vi "CMD_AEROSCRIPTRUN.vi"(6 "Gantry in":refnum<class "Gantry.lvclass">, 8 "error in (no error)":errorcluster, 10 "Arguments":string[](array[string]), 11 "gScript Interpreter in":refnum<class "gScript Interpreter.lvclass">) -> (0 "error out":errorcluster, 3 "gScript Interpreter out":refnum<class "gScript Interpreter.lvclass">, 4 "Gantry out":refnum<class "Gantry.lvclass">)   [LabVIEW 2026, in "gScript Interpreter.lvclass"]
uses:
  gScript Interpreter.lvclass
  Shared Components/Gantry Class/Gantry.lvclass
  Shared Components/FlexWorktable/FlexWorktable.lvclass
  <instrlib>/Aerotech Automation1/Aerotech Automation1.lvlib
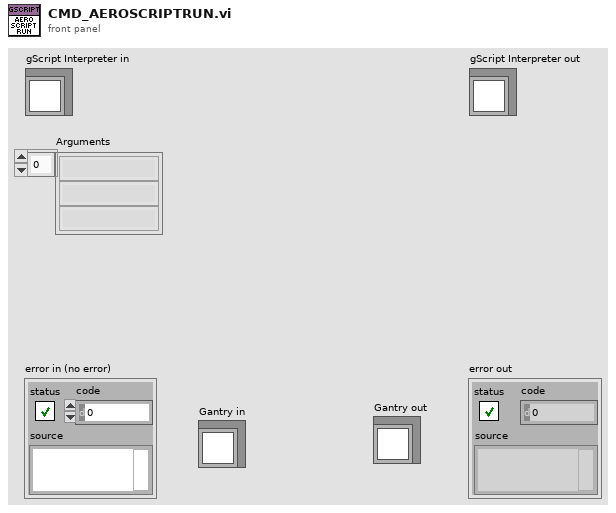
[diagram p1: front panel]
types:
  T1 = enum16{"TLibrary", "T01", "T02", "T03", "T04", "T05", "T06", "T07", "T08", "T09", "T10", "T11", "T12", "T13", "T14", "T15", "T16", "T17", "T18", "T19", "T20", "T21", "T22", "T23", "T24", "T25", "T26", "T27", "T28", "T29", "T30", "T31"}
  T2 = typedef "Virtual Modes.ctl" = enum16{"Nonvirtual", "Virtual"}
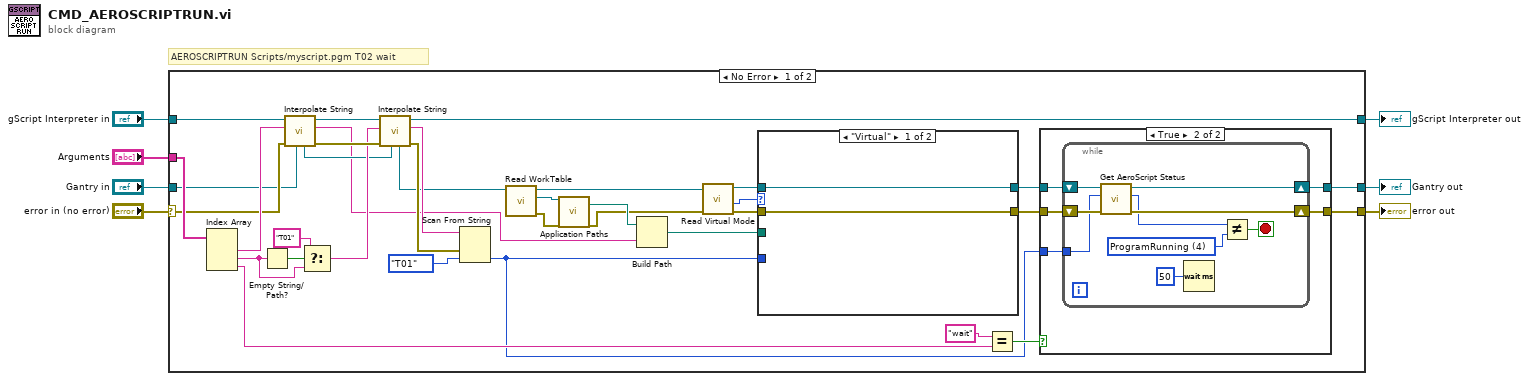
[diagram p0: block diagram]
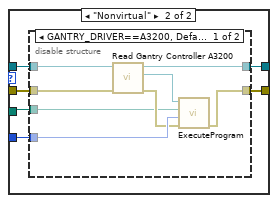
[diagram p3: hidden frame]
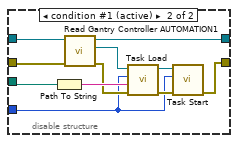
[diagram p4: hidden frame]
diagram:
  # "AEROSCRIPTRUN Scripts/myscript.pgm T02 wait"
  n1 = case shown="No Error" "error in (no error)" {
    selector: "error in (no error)" -> [w39 w88]
    tunnel: [w23 w88] -> w6
    tunnel: [w22 w87] -> w4
    tunnel: "gScript Interpreter in" -> [w41 w87]
    tunnel: "Arguments" -> [w42 _]
    tunnel: "Gantry in" -> [w20 w86]
    tunnel: [w24 w86] -> w1
    frame No Error {
      n2 = Index Array(array=w42) -> (element #1=w40:string, element #2=w33:string, element #3=w29:string)  [unwired: 3 in]
      n3 = Empty String/Path?(string/path=w33) -> (empty?=w34:bool)
      n4 = call-dynamic "Interpolate String.vi"("Gantry in"=w20, "error in (no error)"=w39, "Input String"=w40, "gScript Interpreter in"=w41) -> ("error out"=w37:errorcluster, "Output String"=w10:string, "gScript Interpreter out"=w38:refnum<class "gScript Interpreter.lvclass">, "Gantry out"=w19:refnum<class "Gantry.lvclass">)  [unwired: 4 in]
      n5 = Select(t="T01", s=w34, f=w33) -> (s? t:f=w31:string)
      n6 = call-dynamic "Interpolate String.vi"("Gantry in"=w19, "error in (no error)"=w37, "Input String"=w31, "gScript Interpreter in"=w38) -> ("error out"=w30:errorcluster, "Output String"=w35:string, "gScript Interpreter out"=w22:refnum<class "gScript Interpreter.lvclass">, "Gantry out"=w12:refnum<class "Gantry.lvclass">)  [unwired: 4 in]
      n7 = Scan From String(input string=w35, error in=w30, default 1=T1."T01" ("taskId")) -> (output 1=w21:T1)  [unwired: 2 in, 3 out]
      n8 = call-dynamic "Read WorkTable.vi"("Gantry Class in"=w12) -> ("error out"=w14:errorcluster, "Worktable"=w13:refnum<class "FlexWorktable.lvclass">, "Gantry Class out"=w11:refnum<class "Gantry.lvclass">)  [unwired: 8 in]
      n9 = call "Application Paths.vi"("FlexWorktable in"=w13, "error in (no error)"=w14) -> ("Project Path"=w15:path, "error out"=w9:errorcluster)  [unwired: 11 in, 5 out]
      n10 = Build Path(base path=w15, name or relative path=w10) -> (appended path=w8:path)
      n11 = call-dynamic "Read Virtual Mode.vi"("error in (no error)"=w9, "Gantry in"=w11) -> ("error out"=w17:errorcluster, "Virtual Mode"=w16:T2, "Gantry out"=w18:refnum<class "Gantry.lvclass">)  [unwired: 6 in, 1 out]
      n12 = case shown="\"Virtual\"" w16 {
        tunnel: w17 -> [w59 w63]
        tunnel: [w60 w62] -> w27
        tunnel: [w59 w66] -> w26
        tunnel: w18 -> [w60 w64]
        tunnel: w21 -> [_ w65]
        tunnel: w8 -> [_ w61]
        frame "Virtual" {
        }
        frame "Nonvirtual" {
          n13 = disable-structure shown="GANTRY_DRIVER==A3200, Default" {
            disable-tunnel: [w74 w75] -> w66
            disable-tunnel: w65 -> [w73 w80]
            disable-tunnel: w64 -> [w72 w77]
            disable-tunnel: w63 -> [w71 w78]
            disable-tunnel: [w70 w76] -> w62
            disable-tunnel: w61 -> [w67 w79]
            frame condition #0 {
              n14 = call "Read Gantry Controller A3200.vi"("error in (no error)"=w71, "Gantry in"=w72) -> ("error out"=w68:errorcluster, "A3200 controller out"=w69:refnum<k24>, "Gantry out"=w70:refnum<class "Gantry.lvclass">)  [unwired: 7 in]
              n15 = call "ExecuteProgram.vi"("error in (no error)"=w68, "taskId"=w73, "program name and path"=w67, "controller in"=w69) -> ("error out"=w74:errorcluster)  [unwired: 5 in, 2 out]
            }
            frame condition #1 (active) {
              n16 = Path To String(path=w79) -> (string=w85:string)
              n17 = call "Read Gantry Controller AUTOMATION1.vi"("error in (no error)"=w78, "Gantry in"=w77) -> ("error out"=w83:errorcluster, "Controller AUTOMATION1"=w84:refnum<k24>, "Gantry out"=w76:refnum<class "Gantry.lvclass">)  [unwired: 7 in]
              n18 = call <instrlib>:"Task Load.vi"("error in (no error)"=w83, "Controller Filename"=w85, "Task Index"=w80, "Controller Refnum"=w84) -> ("error out"=w81:errorcluster, "Controller Refnum out"=w82:refnum<k24>)  [unwired: 6 in]
              n19 = call <instrlib>:"Task Start.vi"("error in (no error)"=w81, "Task Index"=w80, "Controller Refnum"=w82) -> ("error out"=w75:errorcluster)  [unwired: 7 in, 1 out]
            }
          }
        }
      }
      n20 = Equal?(x="wait", y=w29) -> (x = y?=w25:bool)
      n21 = case shown="True" w25 {
        tunnel: w27 -> [w44 w49]
        tunnel: w26 -> [w43 w48]
        tunnel: [w44 w47] -> w24
        tunnel: [w43 w46] -> w23
        tunnel: w21 -> [_ w45]
        frame False {
        }
        frame True {
          n22 = while {
            shift-right: [w57] -> w47
            shift-left: w49 -> [w58]
            shift-right: [w55] -> w46
            shift-left: w48 -> [w56]
            tunnel: w45 -> [w54]
            stop <- w52 stop-if-true
            w51 = 4 items=["Unavailable", "Inactive", "Idle", "ProgramReady", "ProgramRunning", "ProgramFeedheld", "ProgramPaused", "ProgramComplete", "Error", "Queue"] ("State")
            n23 = call "Get AeroScript Status.vi"("error in (no error)"=w56, "taskId"=w54, "Gantry in"=w58) -> ("error out"=w55:errorcluster, "State"=w53:i32, "Gantry out"=w57:refnum<class "Gantry.lvclass">)  [unwired: 6 in]
            n24 = Wait (ms)(milliseconds to wait=u32 50) -> ()  [unwired: 1 out]
            n25 = Not Equal?(x=w53, y=w51) -> (x != y?=w52:bool)
          }
        }
      }
    }
    frame Error {
    }
  }
  "error out" <- w6
  "gScript Interpreter out" <- w4
  "Gantry out" <- w1
